vi "Read Timing status.vi"(8 "error in (no error)":errorcluster, 11 "Config params in":refnum<class "CV-Configuration.lvclass">) -> (0 "error out":errorcluster, 2 "Timing status":T1, 3 "Config params out":refnum<class "CV-Configuration.lvclass">)   [LabVIEW 2013, in "CameraVision.lvlib" / "CV-Configuration.lvclass"]
uses:
  CV-Configuration.lvclass
  UI/Module-states.ctl
  CV-Configuration.lvclass/CV-Configuration.ctl
  UI/CV-UI.lvclass
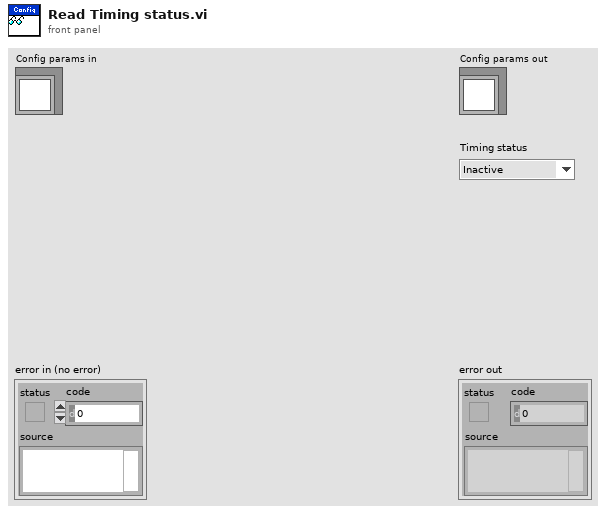
[diagram p1: front panel]
types:
  T1 = typedef "CameraVision.lvlib/CV-UI.lvclass/Module-states.ctl" = enum16{"Inactive", "Active", "Data-loss", "Error", "Simulation", "Synchronizing", "Initialized", "Released"}
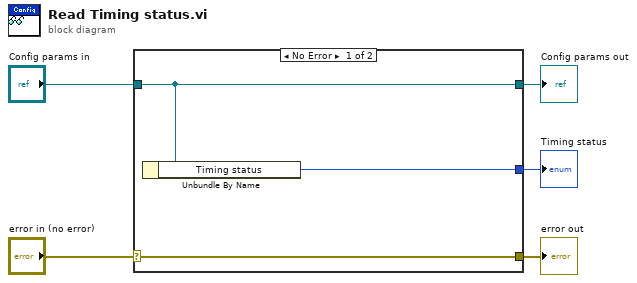
[diagram p0: block diagram]
diagram:
  n1 = case shown="No Error" "error in (no error)" {
    selector: "error in (no error)" -> [w8 w9]
    tunnel: [w8 w9] -> w4
    tunnel: [w7 w10] -> w2
    tunnel: "Config params in" -> [w7 w10]
    tunnel: [w6 _] -> w1
    frame No Error {
      n2 = Unbundle By Name(w7) -> ("Timing status"=w6:T1)
    }
    frame Error {
    }
  }
  "error out" <- w4
  "Config params out" <- w2
  "Timing status" <- w1
